vi "Connect To Path.vi"(0 "Power Meter Base in":refnum<class "Power Meter Base.lvclass">, 5 "DUT Pin":string, 7 "DUT Site":i32, 11 "error in":errorcluster) -> (4 "Power Meter Base out":refnum<class "Power Meter Base.lvclass">, 15 "error out":errorcluster)   [LabVIEW 2023, in "RFFixtureCharact.Instruments.lvlib" / "Power Meter Base.lvclass"]
uses:
  Power Meter Base.lvclass
  Common/RFCalAndFixtureCharact.Common.lvlib
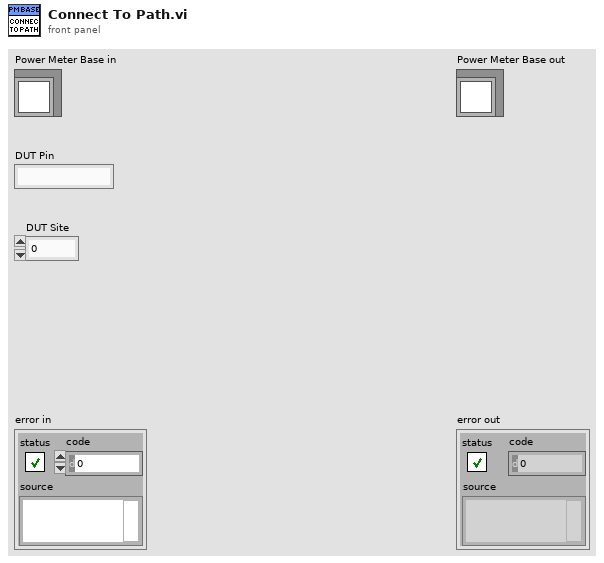
[diagram p1: front panel]
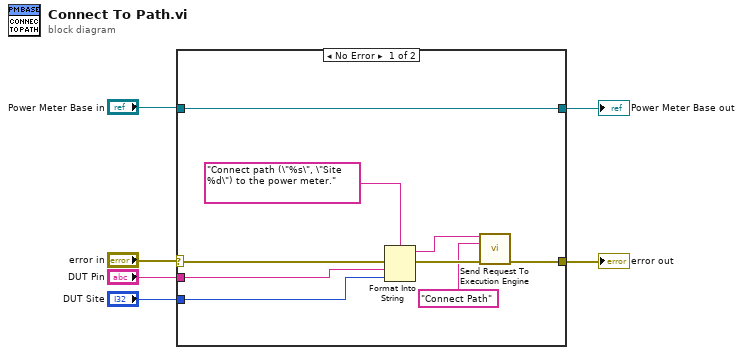
[diagram p0: block diagram]
diagram:
  n1 = case shown="No Error" "error in" {
    selector: "error in" -> [w11 w17]
    tunnel: [w10 w17] -> w4
    tunnel: [w15 w16] -> w3
    tunnel: "Power Meter Base in" -> [w15 w16]
    tunnel: "DUT Site" -> [w8 _]
    tunnel: "DUT Pin" -> [w7 _]
    frame No Error {
      n2 = Format Into String(format string="Connect path (\"%s\", \"Site %d\") to the power meter." ("message"), error in=w11, w7, w8) -> (resulting string=w13:string, error out=w14:errorcluster)  [unwired: 1 in]
      n3 = call "Send Request To Execution Engine.vi"("Request Message"=w13, "Request Header"="Connect Path", "error in (no error)"=w14) -> ("error out"=w10:errorcluster)  [unwired: 11 in, 1 out]
    }
    frame Error {
    }
  }
  "error out" <- w4
  "Power Meter Base out" <- w3
